vi "Axis Selector.vi"(3 "Slave Axis Group":string(combo)="GRPX", 4 "Device Details":T1, 5 "Merc_Ref_Mag In":T2) -> (0 "Slave Present?":bool, 1 "Merc_Ref_Mag Out":T2)   [LabVIEW 2013]
uses:
  <instrlib>/Mercury iXX/Public/Controls/Mercury Reference.ctl
  <instrlib>/Mercury iXX/Public/Controls/Comms Transport Layer.ctl
  <instrlib>/Mercury iXX/Private/Controls/Query Dynamic Reference.ctl
  <instrlib>/Mercury iXX/Mercury iXX.lvlib
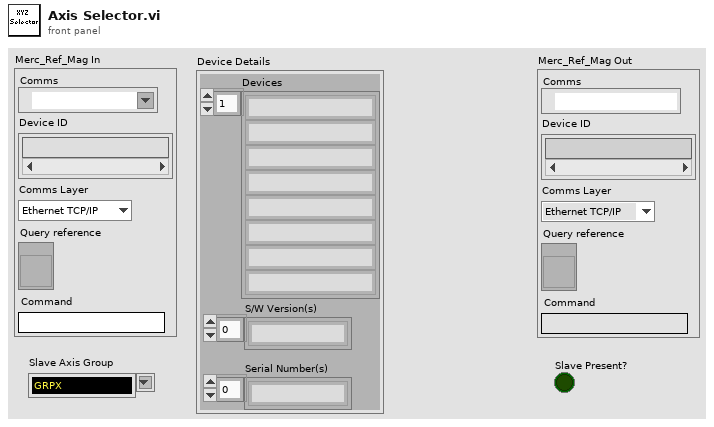
[diagram p1: front panel]
types:
  T1 = cluster{"Devices":string[], "S/W Version(s)":string[], "Serial Number(s)":string[]}
  T2 = typedef "Mercury iXX.lvlib/Mercury Reference.ctl" = cluster{"Comms":refnum<visa-resource-name>, "Device ID":string[], "Comms Layer":T3, "Command":string, "Query reference":T4}
  T3 = typedef "Mercury iXX.lvlib/Comms Transport Layer.ctl" = enum16{"Ethernet TCP/IP", "USB", "ISOBus - RS-232", "GPIB"}
  T4 = typedef "Mercury iXX.lvlib/Query Dynamic Reference.ctl" = refnum<vi>
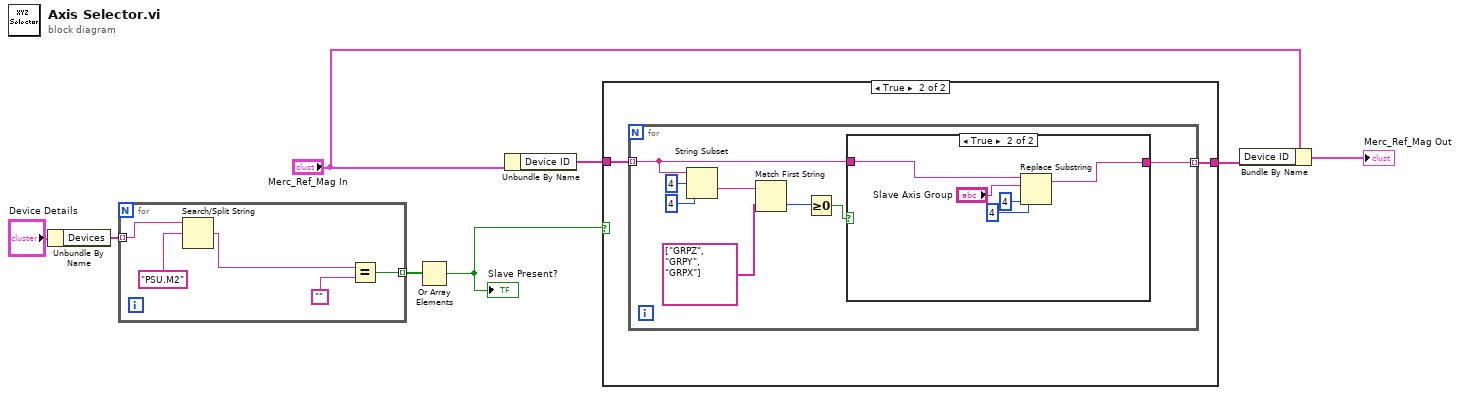
[diagram p0: block diagram]
diagram:
  n1 = Unbundle By Name("Device Details") -> ("Devices"=w3:string[])
  n2 = for {
    tunnel: w3 -> [w13] mode=indexing
    tunnel: [w9] -> w2 mode=indexing
    n3 = Search/Split String(string=w13, search string/char (-)="PSU.M2" ("y")) -> (match + rest of string=w10:string)  [unwired: 1 in, 2 out]
    n4 = Equal?(x=w10, y="") -> (x = y?=w9:bool)
  }
  n5 = Or Array Elements(Boolean array=w2) -> (logical OR=w1:bool)
  "Slave Present?" <- w1
  n6 = Unbundle By Name("Merc_Ref_Mag In") -> ("Device ID"=w8:string[])
  n7 = case shown="True" w1 {
    tunnel: w8 -> [w14 w16]
    tunnel: [w14 w15] -> w6
    frame False {
    }
    frame True {
      n8 = for {
        tunnel: w16 -> [w20] mode=indexing
        tunnel: [w24] -> w15 mode=indexing
        n9 = String Subset(string=w20, offset (0)=4, length (rest)=4 ("length (rest)")) -> (substring=w18:string)
        n10 = Match First String(2:string[] ["GRPZ", "GRPY", "GRPX"], 3:w18) -> (0:w22:i32)  [unwired: 1 out]
        n11 = Greater Or Equal To 0?(x=w22) -> (x >= 0?=w21:bool)
        n12 = case shown="True" w21 {
          tunnel: w20 -> [w25 w30]
          tunnel: [w25 w27] -> w24
          frame False {
          }
          frame True {
            n13 = Replace Substring(2:4 ("length (len. of substring)"), 3:4 ("offset (0)"), 4:"Slave Axis Group", 5:w30) -> (1:w27:string)  [unwired: 1 out]
          }
        }
      }
    }
  }
  n14 = Bundle By Name(cluster="Merc_Ref_Mag In", "Device ID"=w6) -> (→"Merc_Ref_Mag Out":T2)
